vi "Геом прогрессия.vi"(9 "Первый\nчлен":dbl, 10 "Множитель":dbl, 11 "Количество \nЭлеметнов":dbl) -> (2 "Сумма":dbl, 3 "Array":dbl[](array[numeric]))   [LabVIEW 2021]
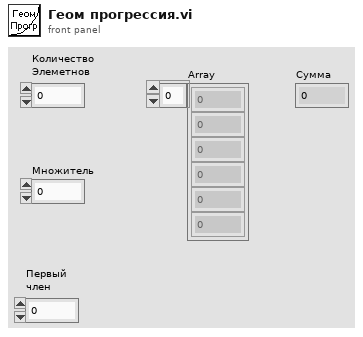
[diagram p1: front panel]
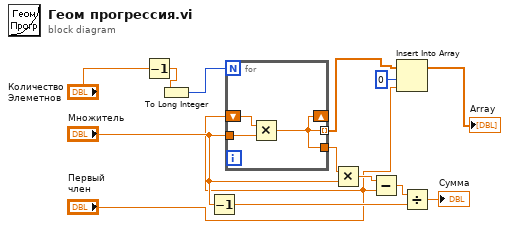
[diagram p0: block diagram]
diagram:
  n1 = Decrement(x="Количество \nЭлеметнов") -> (x-1=w2:dbl)
  n2 = To Long Integer(number=w2) -> (32bit integer=w13:i32)
  n3 = Decrement(x="Множитель") -> (x-1=w8:dbl)
  n4 = for {
    N: w13 -> [_]
    shift-right: [w14] -> _
    shift-left: "Первый\nчлен" -> [w16]
    tunnel: "Множитель" -> [w15]
    tunnel: [w14] -> w4 mode=indexing
    tunnel: [w14] -> w12
    n5 = Multiply(x=w16, y=w15) -> (x*y=w14:dbl)
  }
  n6 = Multiply(x=w12, y="Множитель") -> (x*y=w11:dbl)
  n7 = Subtract(x=w11, y="Первый\nчлен") -> (x-y=w10:dbl)
  n8 = Insert Into Array(array=w4, index=0, new element="Первый\nчлен") -> (→"Array":dbl[])
  n9 = Divide(x=w10, y=w8) -> (x/y=→"Сумма":dbl)
